vi "ReadImageInfo.vi"(8 "error in":errorcluster, 11 "Image Reference In":T2) -> (0 "error out":errorcluster, 1 "Height":i32, 2 "Width":i32, 3 "Image Reference Out":T2, 4 "Image Type":T1, 6 "Image Name":string)   [LabVIEW 2024, in "OpenLvVision_Image.lvlib" / "Management.lvlib"]
doc: "Retrun image information."
uses:
  Management.lvlib
  TypeDef/Image.ctl
  TypeDef/ImageType.ctl
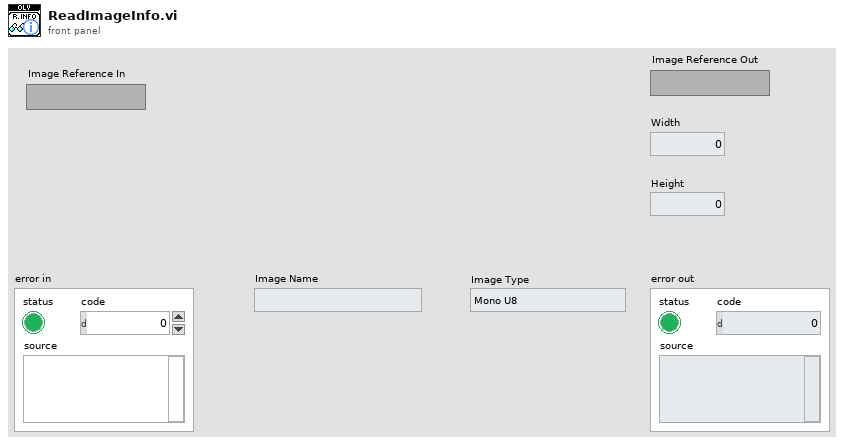
[diagram p1: front panel]
types:
  T1 = typedef "OpenLvVision_Image.lvlib/Management.lvlib/ImageType.ctl" = enum16{"Mono U8", "Mono U16", "Mono I16", "Mono SGL", "Color U32", "Color U64"}
  T2 = typedef "OpenLvVision_Image.lvlib/Management.lvlib/Image.ctl" = refnum<image>
  T3 = typedef "Image Type" = u32
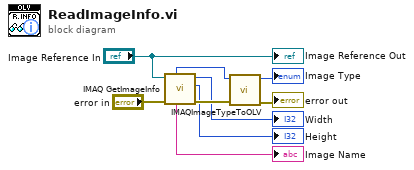
[diagram p0: block diagram]
diagram:
  n1 = call "IMAQ GetImageInfo"("error in (no error)"="error in", "Image"="Image Reference In") -> ("error out"=w6:errorcluster, "Y Resolution"=→"Height":i32, "X Resolution"=→"Width":i32, "Image Name"=→"Image Name":string, "Image Type"=w2:T3)  [unwired: 2 in, 3 out]
  n2 = call "IMAQImageTypeToOLV.vi"("error in"=w6, "IMAQ Image Type"=w2) -> ("error out"=→"error out":errorcluster, "OLV Image Type"=→"Image Type":T1)  [unwired: 8 in]
  "Image Reference Out" <- "Image Reference In"
